vi "CS_PeakDetectionDLL.vi"(6 "PeakSearchParameters":dbl[](array[numeric])=[10.0, 500.0, 3.0, 50.0, 0.3, 0.8, 0.2, 3.0, 2.0], 8 "Error In":errorcluster, 11 "Current Data":T2={"Scan#"=10, "Run Time (mS)"=27811, "TIC X"=[0.0, 0.0515, 0.103, 0.1545, 0.206, 0.25751666666666667, 0.30901666666666666, 0.36051666666666665, 0.41201666666666664, 0.4635166666666667], "TIC Y"=[[210058.0, 491528.0, 394289.0, 802798.0, 237354.0, 91158.0, 8415.0, 4192.0], [220150.0, 493083.0, 399384.0, 808659.0, 236227.0, 86390.0, 8290.0, 3780.0], [217684.0, 490467.0, 390989.0, 794931.0, 229163.0, 83545.0, 7661.0, 3087.0], [210471.0, 478492.0, 378434.0, 773869.0, 210742.0, 74681.0, 5589.0, 1712.0], [187656.0, 432067.0, 325833.0, 674278.0, 159216.0, 51937.0, 3137.0, 769.0], [147176.0, 329962.0, 233061.0, 515895.0, 93836.0, 26991.0, 1305.0, 298.0], [98481.0, 219850.0, 141757.0, 372910.0, 42564.0, 9542.0, 815.0, 185.0], [33487.0, 76569.0, 40250.0, 101775.0, 4294.0, 991.0, 982.0, 309.0], [12052.0, 6742.0, 2362.0, 618.0, 8.0, 2.0, 0.0, 1.0], [4775.0, 6517.0, 2428.0, 647.0, 17.0, 0.0, 0.0, 0.0]], "MassRange"=[{"X Title"="m/z (amu)", "X"=[56.0, 56.1, 56.2, 56.3, 56.4, 56.5, 56.6, 56.7, 56.8, 56.9, 57.0, 57.1, 57.2, 57.3, 57.4, 57.5, 57.6, 57.7, 57.8, 57.9, 58.0, 58.1, 58.2, 58.3, 58.4, 58.5, 58.6, 58.7, 58.8, 58.9, 59.0, 59.1, 59.2, 59.3, 59.4, 59.5, 59.6, 59.7, 59.8, 59.9, 60.0, 60.1, 60.2, 60.3, 60.4, 60.5, 60.6, 60.7, 60.8, 60.9, 61.0, 61.1, 61.2, 61.3, 61.4, 61.5, 61.6, 61.7, 61.8, 61.9, 62.0], "Y"=[202, 289, 353, 348, 294, 441, 1094, 5741, 10137, 18417, 11860, 16848, 14179, 24727, 11093, 10850, 2067, 480, 702, 947, 819, 978, 1319, 2262, 2117, 4148, 14484, 54109, 98223, 158695, 111300, 157540, 127721, 205995, 99332, 97859, 17094, 2902, 3935, 7284, 4697, 6640, 6031, 10313, 4424, 3925, 1473, 288, 510, 677, 443, 725, 625, 776, 464, 474, 209, 22, 26, 44, 19]}, {"X Title"="m/z (amu)", "X"=[114.0, 114.1, 114.2, 114.3, 114.4, 114.5, 114.6, 114.7, 114.8, 114.9, 115.0, 115.1, 115.2, 115.3, 115.4, 115.5, 115.6, 115.7, 115.8, 115.9, 116.0, 116.1, 116.2, 116.3, 116.4, 116.5, 116.6, 116.7, 116.8, 116.9, 117.0, 117.1, 117.2, 117.3, 117.4, 117.5, 117.6, 117.7, 117.8, 117.9, 118.0, 118.1, 118.2, 118.3, 118.4, 118.5, 118.6, 118.7, 118.8, 118.9, 119.0, 119.1, 119.2, 119.3, 119.4, 119.5, 119.6, 119.7, 119.8, 119.9, 120.0], "Y"=[491, 489, 596, 954, 6594, 10175, 11103, 24346, 24112, 21758, 47429, 24868, 33806, 24592, 32419, 10316, 2688, 3358, 3320, 4390, 5939, 4445, 5547, 8057, 37094, 125620, 138850, 227250, 245109, 221731, 292773, 234264, 267655, 245559, 276939, 113302, 17927, 26519, 21182, 19895, 37275, 29365, 26177, 26351, 38186, 13114, 2386, 2759, 2618, 2661, 5309, 2754, 3952, 2975, 3512, 1047, 343, 201, 233, 235, 363]}, {"X Title"="m/z (amu)", "X"=[172.0, 172.1, 172.2, 172.3, 172.4, 172.5, 172.6, 172.7, 172.8, 172.9, 173.0, 173.1, 173.2, 173.3, 173.4, 173.5, 173.6, 173.7, 173.8, 173.9, 174.0, 174.1, 174.2, 174.3, 174.4, 174.5, 174.6, 174.7, 174.8, 174.9, 175.0, 175.1, 175.2, 175.3, 175.4, 175.5, 175.6, 175.7, 175.8, 175.9, 176.0, 176.1, 176.2, 176.3, 176.4, 176.5, 176.6, 176.7, 176.8, 176.9, 177.0, 177.1, 177.2, 177.3, 177.4, 177.5, 177.6, 177.7, 177.8, 177.9, 178.0], "Y"=[207, 219, 342, 749, 2242, 3102, 3875, 4753, 6787, 6179, 9971, 6402, 10854, 6982, 6994, 2894, 1160, 1376, 1525, 1703, 2474, 1831, 3750, 18133, 44833, 81418, 111480, 141238, 191269, 183454, 245368, 181046, 246802, 191469, 199038, 80459, 23328, 20529, 26315, 25338, 36487, 26534, 31775, 28885, 32358, 12210, 4849, 2880, 4053, 3672, 5595, 3672, 6431, 4058, 3885, 1440, 356, 330, 417, 420, 592]}, {"X Title"="m/z (amu)", "X"=[381.0, 381.1, 381.2, 381.3, 381.4, 381.5, 381.6, 381.7, 381.8, 381.9, 382.0, 382.1, 382.2, 382.3, 382.4, 382.5, 382.6, 382.7, 382.8, 382.9, 383.0, 383.1, 383.2, 383.3, 383.4, 383.5, 383.6, 383.7, 383.8, 383.9, 384.0, 384.1, 384.2, 384.3, 384.4, 384.5, 384.6, 384.7, 384.8, 384.9, 385.0, 385.1, 385.2, 385.3, 385.4, 385.5, 385.6, 385.7, 385.8, 385.9, 386.0, 386.1, 386.2, 386.3, 386.4, 386.5, 386.6, 386.7, 386.8, 386.9, 387.0], "Y"=[5350, 5975, 6890, 8616, 9486, 10258, 11035, 10226, 13126, 12765, 10852, 15551, 13397, 13198, 10338, 8901, 7501, 6912, 7299, 7131, 11259, 36335, 75636, 121474, 175491, 215134, 245501, 252477, 268512, 282567, 258781, 292901, 282509, 287557, 227968, 214745, 174181, 144936, 123295, 111476, 82903, 103746, 104923, 102997, 72674, 64365, 43455, 34237, 30361, 23734, 19110, 25135, 22272, 23982, 20150, 16952, 13814, 12183, 11344, 11504, 8997]}, {"X Title"="m/z (amu)", "X"=[613.0, 613.1, 613.2, 613.3, 613.4, 613.5, 613.6, 613.7, 613.8, 613.9, 614.0, 614.1, 614.2, 614.3, 614.4, 614.5, 614.6, 614.7, 614.8, 614.9, 615.0, 615.1, 615.2, 615.3, 615.4, 615.5, 615.6, 615.7, 615.8, 615.9, 616.0, 616.1, 616.2, 616.3, 616.4, 616.5, 616.6, 616.7, 616.8, 616.9, 617.0, 617.1, 617.2, 617.3, 617.4, 617.5, 617.6, 617.7, 617.8, 617.9, 618.0, 618.1, 618.2, 618.3, 618.4, 618.5, 618.6, 618.7, 618.8, 618.9, 619.0], "Y"=[871, 910, 877, 832, 811, 881, 824, 887, 1018, 1368, 1586, 1608, 1601, 1951, 2007, 2146, 2220, 2153, 2297, 2721, 2965, 3304, 4167, 4917, 7038, 11211, 17183, 24096, 33872, 40149, 55165, 60024, 68766, 82553, 79641, 86329, 80741, 63103, 43494, 36766, 35876, 36007, 36976, 35568, 31109, 32133, 29192, 25845, 16843, 12613, 11138, 10411, 10403, 10339, 8702, 8717, 8391, 6149, 4561, 3659, 3736]}, {"X Title"="m/z (amu)", "X"=[904.0, 904.1, 904.2, 904.3, 904.4, 904.5, 904.6, 904.7, 904.8, 904.9, 905.0, 905.1, 905.2, 905.3, 905.4, 905.5, 905.6, 905.7, 905.8, 905.9, 906.0, 906.1, 906.2, 906.3, 906.4, 906.5, 906.6, 906.7, 906.8, 906.9, 907.0, 907.1, 907.2, 907.3, 907.4, 907.5, 907.6, 907.7, 907.8, 907.9, 908.0, 908.1, 908.2, 908.3, 908.4, 908.5, 908.6, 908.7, 908.8, 908.9, 909.0, 909.1, 909.2, 909.3, 909.4, 909.5, 909.6, 909.7, 909.8, 909.9, 910.0], "Y"=[1326, 1563, 1907, 2126, 2287, 2590, 2612, 2688, 2653, 2481, 2145, 2103, 2256, 2141, 2699, 2961, 3890, 4835, 6292, 8338, 9675, 12116, 14336, 16870, 18680, 19689, 21074, 20694, 20138, 17909, 12631, 11561, 11287, 11387, 11909, 12243, 12764, 12111, 11520, 10216, 7314, 5603, 5495, 5280, 5274, 5491, 5264, 5137, 4830, 4128, 2799, 2467, 2238, 2260, 2087, 2125, 2166, 1928, 1695, 1644, 1309]}, {"X Title"="m/z (amu)", "X"=[1542.0, 1542.1, 1542.2, 1542.3, 1542.4, 1542.5, 1542.6, 1542.7, 1542.8, 1542.9, 1543.0, 1543.1, 1543.2, 1543.3, 1543.4, 1543.5, 1543.6, 1543.7, 1543.8, 1543.9, 1544.0, 1544.1, 1544.2, 1544.3, 1544.4, 1544.5, 1544.6, 1544.7, 1544.8, 1544.9, 1545.0, 1545.1, 1545.2, 1545.3, 1545.4, 1545.5, 1545.6, 1545.7, 1545.8, 1545.9, 1546.0, 1546.1, 1546.2, 1546.3, 1546.4, 1546.5, 1546.6, 1546.7, 1546.8, 1546.9, 1547.0, 1547.1, 1547.2, 1547.3, 1547.4, 1547.5, 1547.6, 1547.7, 1547.8, 1547.9, 1548.0], "Y"=[125, 143, 166, 163, 155, 150, 181, 180, 161, 177, 176, 239, 187, 207, 214, 229, 263, 244, 305, 370, 452, 505, 593, 683, 722, 781, 1023, 1088, 1217, 1202, 1279, 1225, 1082, 968, 953, 943, 950, 1012, 1102, 1196, 1111, 1028, 933, 846, 691, 685, 595, 703, 697, 727, 702, 671, 563, 507, 453, 440, 348, 419, 367, 357, 340]}, {"X Title"="m/z (amu)", "X"=[2007.0, 2007.1, 2007.2, 2007.3, 2007.4, 2007.5, 2007.6, 2007.7, 2007.8, 2007.9, 2008.0, 2008.1, 2008.2, 2008.3, 2008.4, 2008.5, 2008.6, 2008.7, 2008.8, 2008.9, 2009.0, 2009.1, 2009.2, 2009.3, 2009.4, 2009.5, 2009.6, 2009.7, 2009.8, 2009.9, 2010.0, 2010.1, 2010.2, 2010.3, 2010.4, 2010.5, 2010.6, 2010.7, 2010.8, 2010.9, 2011.0, 2011.1, 2011.2, 2011.3, 2011.4, 2011.5, 2011.6, 2011.7, 2011.8, 2011.9, 2012.0, 2012.1, 2012.2, 2012.3, 2012.4, 2012.5, 2012.6, 2012.7, 2012.8, 2012.9, 2013.0], "Y"=[72, 58, 44, 62, 33, 40, 37, 55, 40, 65, 42, 41, 38, 66, 69, 76, 53, 62, 66, 94, 133, 128, 126, 146, 265, 258, 342, 380, 421, 574, 565, 647, 692, 720, 696, 603, 545, 525, 493, 476, 395, 438, 361, 390, 318, 273, 267, 239, 249, 214, 183, 199, 163, 119, 122, 127, 111, 86, 91, 58, 82]}], "Fixed Mass (amu)"=609.2, "Method"={"StartT(mS)"=0, "#Cycles"=10, "PauseT(uS)"=5000, "ScanType"=1, "Polarity"=0, "FixedMass"=609.2, "DelayT(mS)"=0, "Active Ch"=[{"Value"=400.0, "ChID"=1}, {"Value"=600.0, "ChID"=4}, {"Value"=32768.0, "ChID"=7}, {"Value"=400.0, "ChID"=2}, {"Value"=600.0, "ChID"=5}, {"Value"=32768.0, "ChID"=9}, {"Value"=450.0, "ChID"=3}, {"Value"=0.0, "ChID"=20}, {"Value"=0.0, "ChID"=21}, {"Value"=0.0, "ChID"=19}, {"Value"=0.0, "ChID"=18}, {"Value"=0.0, "ChID"=22}, {"Value"=0.0, "ChID"=11}, {"Value"=-20.0, "ChID"=12}, {"Value"=-2.0, "ChID"=6}, {"Value"=0.0, "ChID"=13}, {"Value"=-180.0, "ChID"=14}, {"Value"=-50.0, "ChID"=23}, {"Value"=100.0, "ChID"=10}, {"Value"=-200.0, "ChID"=15}, {"Value"=-200.0, "ChID"=16}, {"Value"=-52.0, "ChID"=8}, {"Value"=-100.0, "ChID"=17}, {"Value"=15.0, "ChID"=32}, {"Value"=2200.0, "ChID"=34}, {"Value"=5500.0, "ChID"=200}, {"Value"=420.0, "ChID"=36}, {"Value"=-420.0, "ChID"=37}, {"Value"=420.0, "ChID"=38}, {"Value"=-420.0, "ChID"=39}, {"Value"=600.0, "ChID"=40}, {"Value"=-600.0, "ChID"=41}, {"Value"=60.0, "ChID"=26}, {"Value"=110.0, "ChID"=27}, {"Value"=0.0, "ChID"=29}, {"Value"=0.0, "ChID"=28}, {"Value"=0.0, "ChID"=30}, {"Value"=0.0, "ChID"=43}, {"Value"=500.0, "ChID"=42}, {"Value"=0.0, "ChID"=204}, {"Value"=5200.0, "ChID"=203}, {"Value"=0.0, "ChID"=202}, {"Value"=1000.0, "ChID"=201}, {"Value"=320.0, "ChID"=81}, {"Value"=0.0, "ChID"=86}, {"Value"=0.0, "ChID"=84}], "Mass Range"=[{"Start"=56.0, "Stop"=62.0, "Step Size"=0.1, "Steps"=61, "Dwell"=5.0, "Parameters"=[{"Name"="EV", "Ch#"=20, "StartV"=55.0, "StopV"=55.0, "StepV"=0.0, "Index"=7}], "Res"=1}, {"Start"=114.0, "Stop"=120.0, "Step Size"=0.1, "Steps"=61, "Dwell"=5.0, "Parameters"=[{"Name"="EV", "Ch#"=20, "StartV"=55.0, "StopV"=55.0, "StepV"=0.0, "Index"=7}], "Res"=1}, {"Start"=172.0, "Stop"=178.0, "Step Size"=0.1, "Steps"=61, "Dwell"=5.0, "Parameters"=[{"Name"="EV", "Ch#"=20, "StartV"=55.0, "StopV"=55.0, "StepV"=0.0, "Index"=7}], "Res"=1}, {"Start"=381.0, "Stop"=387.0, "Step Size"=0.1, "Steps"=61, "Dwell"=5.0, "Parameters"=[{"Name"="EV", "Ch#"=20, "StartV"=0.0, "StopV"=0.0, "StepV"=0.0, "Index"=7}], "Res"=1}, {"Start"=613.0, "Stop"=619.0, "Step Size"=0.1, "Steps"=61, "Dwell"=5.0, "Parameters"=[{"Name"="EV", "Ch#"=20, "StartV"=55.0, "StopV"=55.0, "StepV"=0.0, "Index"=7}], "Res"=1}, {"Start"=904.0, "Stop"=910.0, "Step Size"=0.1, "Steps"=61, "Dwell"=5.0, "Parameters"=[{"Name"="EV", "Ch#"=20, "StartV"=55.0, "StopV"=55.0, "StepV"=0.0, "Index"=7}], "Res"=1}, {"Start"=1542.0, "Stop"=1548.0, "Step Size"=0.1, "Steps"=61, "Dwell"=10.0, "Parameters"=[{"Name"="EV", "Ch#"=20, "StartV"=70.0, "StopV"=70.0, "StepV"=0.0, "Index"=7}], "Res"=1}, {"Start"=2007.0, "Stop"=2013.0, "Step Size"=0.1, "Steps"=61, "Dwell"=10.0, "Parameters"=[{"Name"="EV", "Ch#"=20, "StartV"=55.0, "StopV"=55.0, "StepV"=0.0, "Index"=7}], "Res"=1}]}} {"Method"."Mass Range"."Res" items=["High/High", "Medium/Medium", "Low/Low", "High/Medium", "High/Low", "Medium/High", "Medium/Low", "Low/High", "Low/Medium"]}) -> (0 "Error Out":errorcluster, 3 "Peak List":T1[](array[typedef]))   [LabVIEW 2015]
uses:
  Type/_Current Data.ctl
  Type/_XML Expt.ctl
  Type/_XML Lens.ctl
  Type/_Mass Range Property.ctl
  Type/_Mass Range Parameters.ctl
  Type/_RT Res Type.ctl
  Type/_Peak Property.ctl
  C:/GitRepo/PerkinElmer/EH-Qfirmwareserver/firmware-server/Sniffer.900/External Dependencies/PerkinElmer.SimplicityServer.LVWrapper.dll
  External Dependencies/PerkinElmer.SimplicityServer.LVWrapper.dll
panel:
  # "MinimumMassPeakWidth"
  # "0"
  # "ThresholdForMassSpectrum"
  # "1"
  # "2"
  # "SearchRange"
  # "WidthAtOfMaximum"
  # "5"
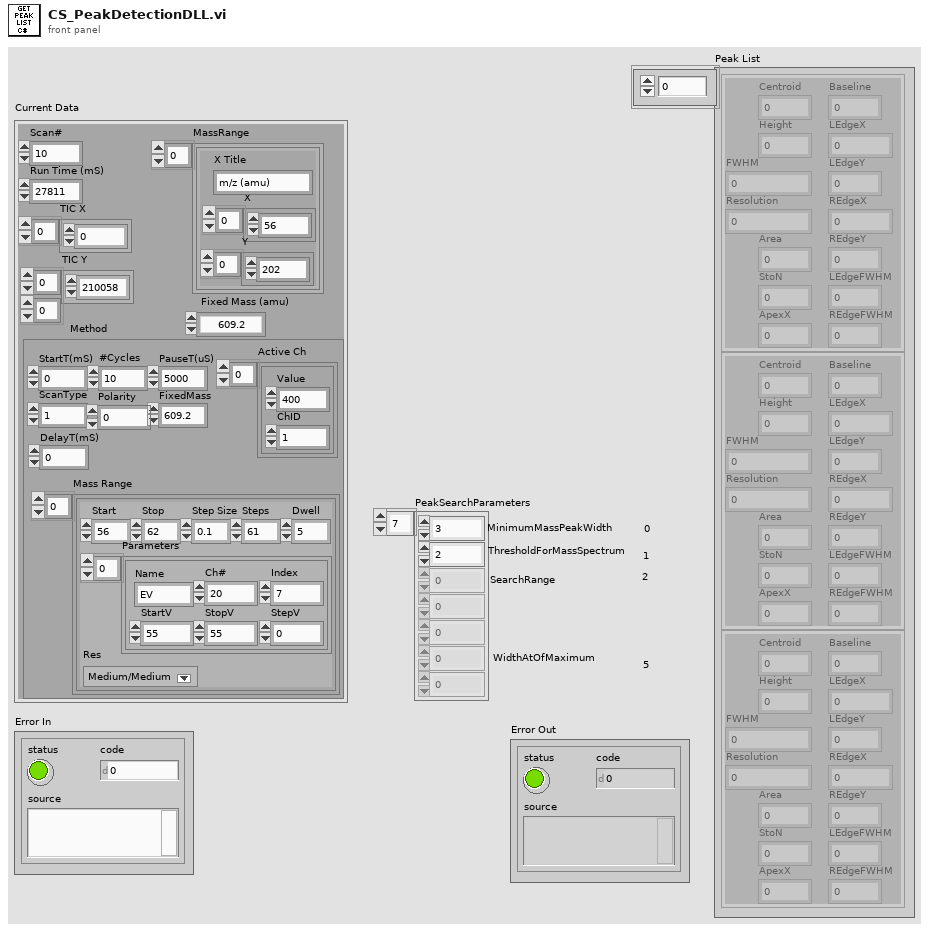
[diagram p1: front panel]
types:
  T1 = typedef "_Peak Property.ctl" = cluster{"Centroid":dbl, "Height":dbl, "FWHM":dbl, "Resolution":dbl, "Area":dbl, "StoN":dbl, "ApexX":dbl, "Baseline":dbl, "LEdgeX":dbl, "LEdgeY":dbl, "REdgeX":dbl, "REdgeY":dbl, "LEdgeFWHM":dbl, "REdgeFWHM":dbl}
  T2 = typedef "_Current Data.ctl" = cluster{"Scan#":i32, "Run Time (mS)":i32, "TIC X":dbl[], "TIC Y":dbl[][], "MassRange":cluster{"X Title":string, "X":dbl[], "Y":i32[]}[], "Fixed Mass (amu)":dbl, "Method":T3}
  T3 = typedef "_XML Expt.ctl" = cluster{"StartT(mS)":i32, "#Cycles":i32, "PauseT(uS)":i32, "ScanType":i32, "Polarity":u8, "FixedMass":dbl, "DelayT(mS)":i32, "Active Ch":T4[], "Mass Range":T5[]}
  T4 = typedef "_XML Lens.ctl" = cluster{"Value":dbl, "ChID":u8}
  T5 = typedef "_Mass Range Property.ctl" = cluster{"Start":dbl, "Stop":dbl, "Step Size":dbl, "Steps":i32, "Dwell":dbl, "Parameters":T6[], "Res":T7}
  T6 = typedef "_Mass Range Parameters.ctl" = cluster{"Name":string, "Ch#":u8, "StartV":dbl, "StopV":dbl, "StepV":dbl, "Index":u8}
  T7 = typedef "_RT Res Type.ctl" = u16
  T8 = cluster{"X Title":string, "X":dbl[], "Y":i32[]}[]
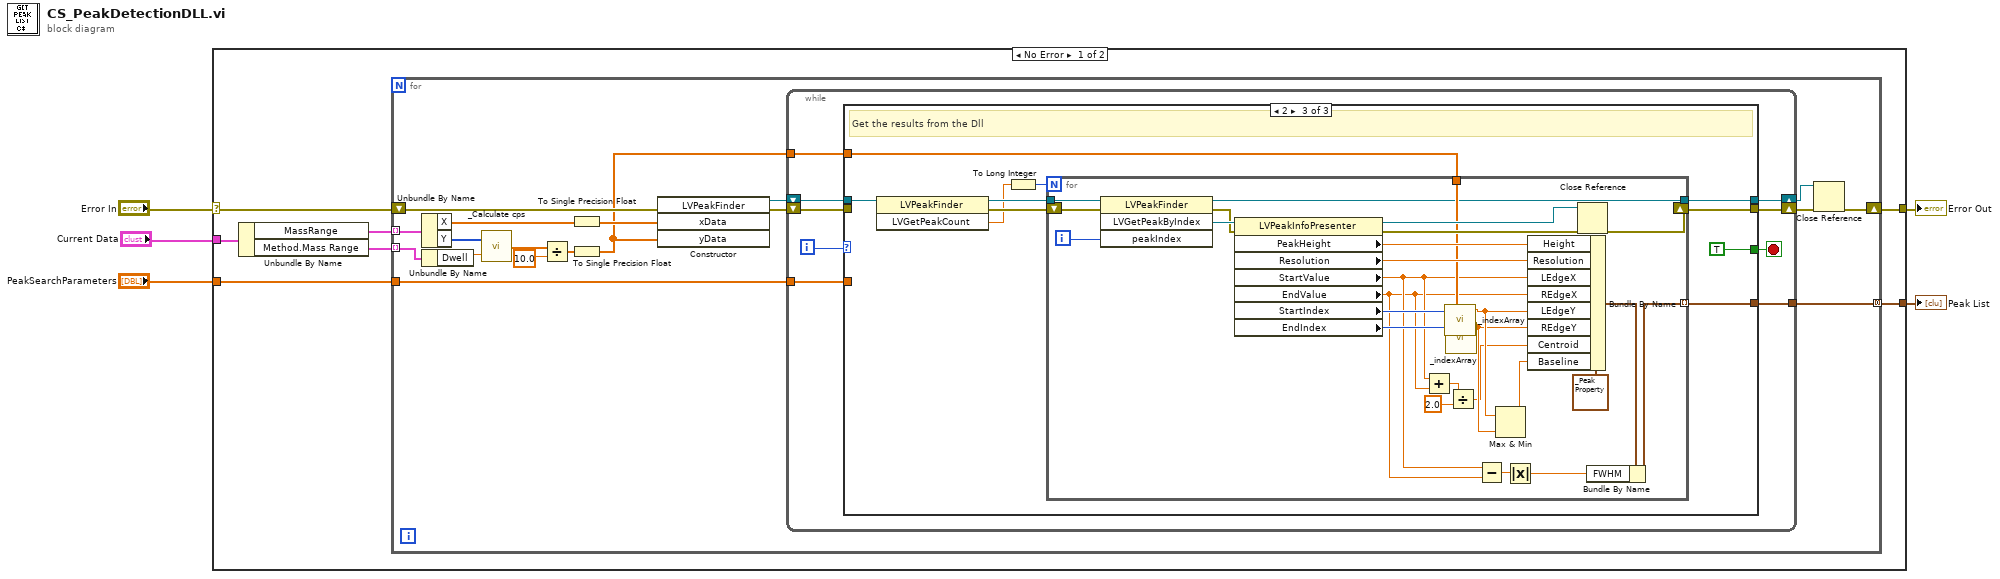
[diagram p0: block diagram]
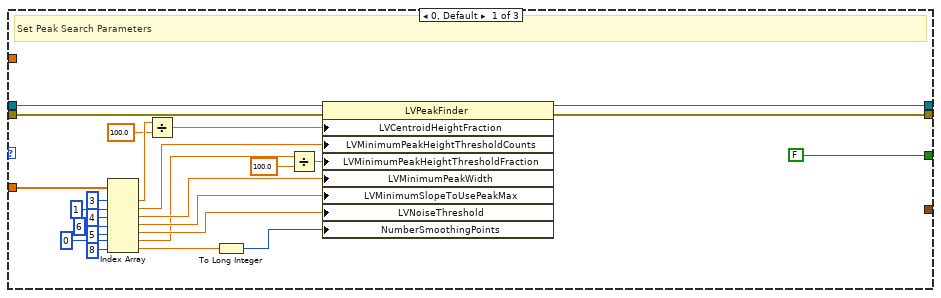
[diagram p2: hidden frame]
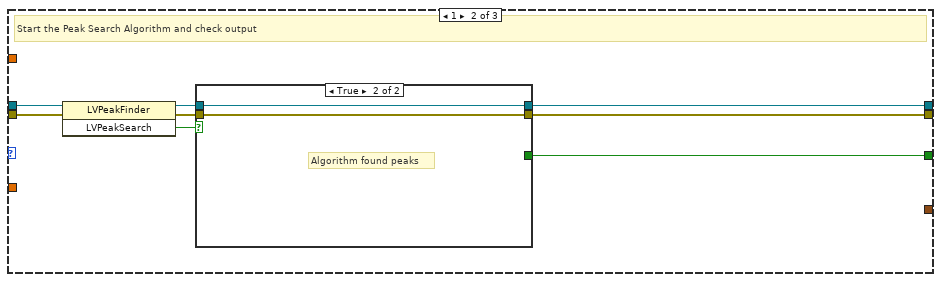
[diagram p3: hidden frame]
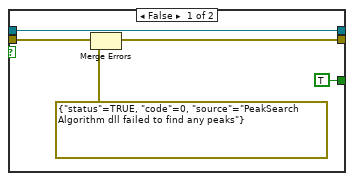
[diagram p4: hidden frame]
diagram:
  n1 = case shown="No Error" "Error In" {
    selector: "Error In" -> [w8 w117]
    tunnel: "Current Data" -> [w12 _]
    tunnel: "PeakSearchParameters" -> [w9 _]
    tunnel: [w7 w117] -> w2
    tunnel: [w6 _] -> w1
    frame No Error {
      n2 = Unbundle By Name(w12) -> ("MassRange"=w11:T8, "Method.Mass Range"=w10:T5[])
      n3 = for {
        tunnel: w11 -> [w26] mode=indexing
        tunnel: w10 -> [w27] mode=indexing
        tunnel: w9 -> [w23]
        shift-right: [w20] -> w7
        shift-left: w8 -> [w15]
        tunnel: [w18] -> w6 mode=concatenating
        n4 = Unbundle By Name(w26) -> ("X"=w22:dbl[], "Y"=w25:i32[])
        n5 = Unbundle By Name(w27) -> ("Dwell"=w28:dbl)
        n6 = call "_Calculate cps.vi"("Dwell (mS)"=w28, "Raw Counts"=w25) -> ("Data in cps"=w29:dbl[])
        n7 = Divide(x=w29, y=10.0) -> (x/y=w24:dbl[])
        n8 = To Single Precision Float(number=w22) -> (single precision float=w14:sgl[])
        n9 = To Single Precision Float(number=w24) -> (single precision float=w13:sgl[])
        n10 = constructor class="LVPeakFinder"(error in=w15, "xData"=w14, "yData"=w13) -> (reference out=w17:refnum<k24>, error out=w16:errorcluster)  [unwired: 2 in, 3 out]
        n11 = while {
          shift-right: [w33] -> w19
          shift-left: w17 -> [w36]
          tunnel: w23 -> [w39]
          shift-right: [w34] -> w21
          shift-left: w16 -> [w37]
          tunnel: [w32] -> w18
          tunnel: w13 -> [w35]
          i -> [w38]
          stop <- w31 stop-if-true
          n12 = case shown="2" w38 {
            tunnel: w37 -> [w64 w71 _]
            tunnel: w36 -> [w63 w72 w80]
            tunnel: [w62 w70 w88] -> w33
            tunnel: w39 -> [w61 _ _]
            tunnel: [w59 w67 w87] -> w34
            tunnel: [FALSE w65 TRUE] -> w31
            tunnel: [_ _ w86] -> w32
            tunnel: w35 -> [_ _ w84]
            frame 0, Default {
              # "Set Peak Search Parameters"
              n13 = Index Array(array=w61, index #1=3 ("index"), index #2=1 ("index"), index #3=4 ("index"), index #4=6 ("index"), index #5=5 ("index"), index #6=0 ("index"), index #7=8 ("index")) -> (element #1=w57:dbl, element #2=w55:dbl, element #3=w53:dbl, element #4=w51:dbl, element #5=w49:dbl, element #6=w47:dbl, element #7=w41:dbl)
              n14 = Divide(x=w57, y=100.0 ("x")) -> (x/y=w46:dbl)
              n15 = To Long Integer(number=w41) -> (32bit integer=w40:i32)
              n16 = Divide(x=w47, y=100.0 ("x")) -> (x/y=w44:dbl)
              n17 = property class="LVPeakFinder"(reference=w63, error in=w64, "LVCentroidHeightFraction"=w46, "LVMinimumPeakHeightThresholdCounts"=w55, "LVMinimumPeakHeightThresholdFraction"=w44, "LVMinimumPeakWidth"=w53, "LVMinimumSlopeToUsePeakMax"=w51, "LVNoiseThreshold"=w49, "NumberSmoothingPoints"=w40) -> (reference out=w62:refnum<k24>, error out=w59:errorcluster)
            }
            frame 1 {
              # "Start the Peak Search Algorithm and check output"
              n18 = invoke class="LVPeakFinder" method="LVPeakSearch"(reference=w72, error in=w71) -> (reference out=w69:refnum<k24>, error out=w68:errorcluster, "LVPeakSearch"=w66:bool)  [unwired: 1 in]
              n19 = case shown="True" w66 {
                tunnel: [w77 w79] -> w70
                tunnel: w69 -> [w77 w79]
                tunnel: w68 -> [w76 w78]
                tunnel: [w74 w78] -> w67
                tunnel: [TRUE _] -> w65
                frame False {
                  n20 = Merge Errors(errorcluster {"status"=TRUE, "code"=0, "source"="PeakSearch Algorithm dll failed to find any peaks"} ("error in"), w76) -> (w74:errorcluster)
                }
                frame True {
                  # "Algorithm found peaks"
                }
              }
            }
            frame 2 {
              # "Get the results from the Dll"
              n21 = invoke class="LVPeakFinder" method="LVGetPeakCount"(reference=w80) -> (reference out=w89:refnum<k24>, error out=w83:errorcluster, "LVGetPeakCount"=w82:dbl)  [unwired: 2 in]
              n22 = To Long Integer(number=w82) -> (32bit integer=w81:i32)
              n23 = for {
                N: w81 -> [_]
                tunnel: [w94] -> w88
                tunnel: w89 -> [w90]
                shift-right: [w111] -> w87
                shift-left: w83 -> [w95]
                tunnel: [w108] -> w86 mode=indexing
                tunnel: w84 -> [w107]
                i -> [w93]
                n24 = invoke class="LVPeakFinder" method="LVGetPeakByIndex"(reference=w90, error in=w95, "peakIndex"=w93) -> (reference out=w94:refnum<k24>, error out=w91:errorcluster, "LVGetPeakByIndex"=w92:refnum<k24>)  [unwired: 1 in, 1 out]
                n25 = property class="LVPeakInfoPresenter"(reference=w92, error in=w91) -> (reference out=w112:refnum<k24>, error out=w113:errorcluster, "PeakHeight"=w115:dbl, "Resolution"=w114:dbl, "StartValue"=w100:dbl, "EndValue"=w99:dbl, "StartIndex"=w104:i32, "EndIndex"=w103:i32)
                n26 = Add(x=w100, y=w99) -> (x+y=w98:dbl)
                n27 = call "_indexArray.vi"("xData"=w107, "index"=w104) -> ("Data Point"=w106:dbl)  [unwired: 9 in]
                n28 = call "_indexArray.vi"("xData"=w107, "index"=w103) -> ("Data Point"=w105:dbl)  [unwired: 9 in]
                n29 = Divide(x=w98, y=2.0) -> (x/y=w96:dbl)
                n30 = Subtract(x=w100, y=w99) -> (x-y=w102:dbl)
                n31 = Max & Min(x=w106, y=w105) -> (min(x,y)=w110:dbl)  [unwired: 1 out]
                n32 = Absolute Value(x=w102) -> (abs(x)=w101:dbl)
                n33 = Bundle By Name(cluster=T1 {"Centroid"=0.0, "Height"=0.0, "FWHM"=0.0, "Resolution"=0.0, "Area"=0.0, "StoN"=0.0, "ApexX"=0.0, "Baseline"=0.0, "LEdgeX"=0.0, "LEdgeY"=0.0, "REdgeX"=0.0, "REdgeY"=0.0, "LEdgeFWHM"=0.0, "REdgeFWHM"=0.0} ("Peak"), "Height"=w115, "Resolution"=w114, "LEdgeX"=w100, "REdgeX"=w99, "LEdgeY"=w106, "REdgeY"=w105, "Centroid"=w96, "Baseline"=w110) -> (w109:T1)
                n34 = Close Reference(reference=w112, error in (no error)=w113) -> (error out=w111:errorcluster)
                n35 = Bundle By Name(cluster=w109, "FWHM"=w101) -> (w108:T1)
              }
            }
          }
        }
        n36 = Close Reference(reference=w19, error in (no error)=w21) -> (error out=w20:errorcluster)
      }
    }
    frame Error {
    }
  }
  "Error Out" <- w2
  "Peak List" <- w1
